vi "mono_rpm.vi"(7 "Sensor Connections":T1(array[cluster])) -> (0 "error out":errorcluster, 1 "wheel_rpm_sample":T2, 2 "Sensor Connections Out":T1(array[cluster]), 3 "tcp_out":refnum<k5>)   [LabVIEW 2018, in "monoDrive.lvlib"]
uses:
  monoDrive.lvlib
panel:
  in  "wheel_speed_rr":u8
  in  "wheel_speed_lr":u8
  in  "wheel_speed_rf":u8
  in  "wheel_speed_lf":u8
  in  "wheel_number":u32
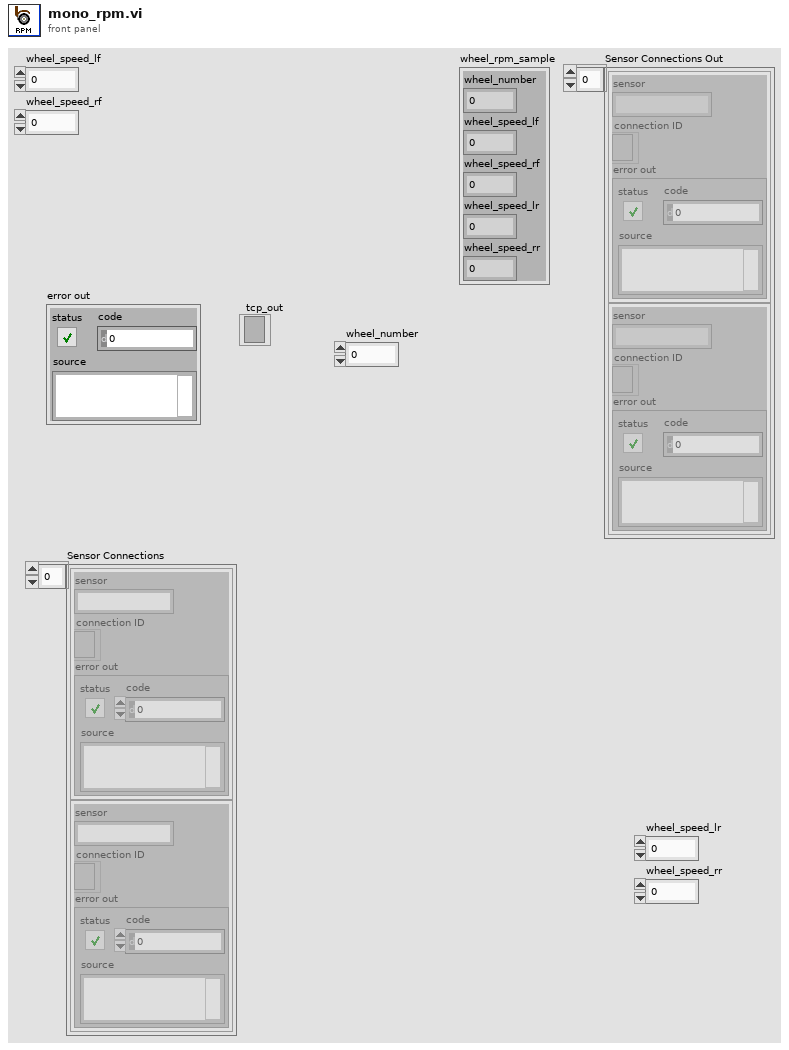
[diagram p1: front panel]
types:
  T1 = cluster{"sensor":string, "connection ID":refnum<k5>, "error out":errorcluster}[]
  T2 = cluster{"wheel_number":u32, "wheel_speed_lf":u8, "wheel_speed_rf":u8, "wheel_speed_lr":u8, "wheel_speed_rr":u8}
  T3 = cluster{"sensor":string, "connection ID":refnum<k5>, "error out":errorcluster}
  T4 = cluster{cluster{"length":u32, "time_stamp":u32, "game_time":sgl}, "data out":string}
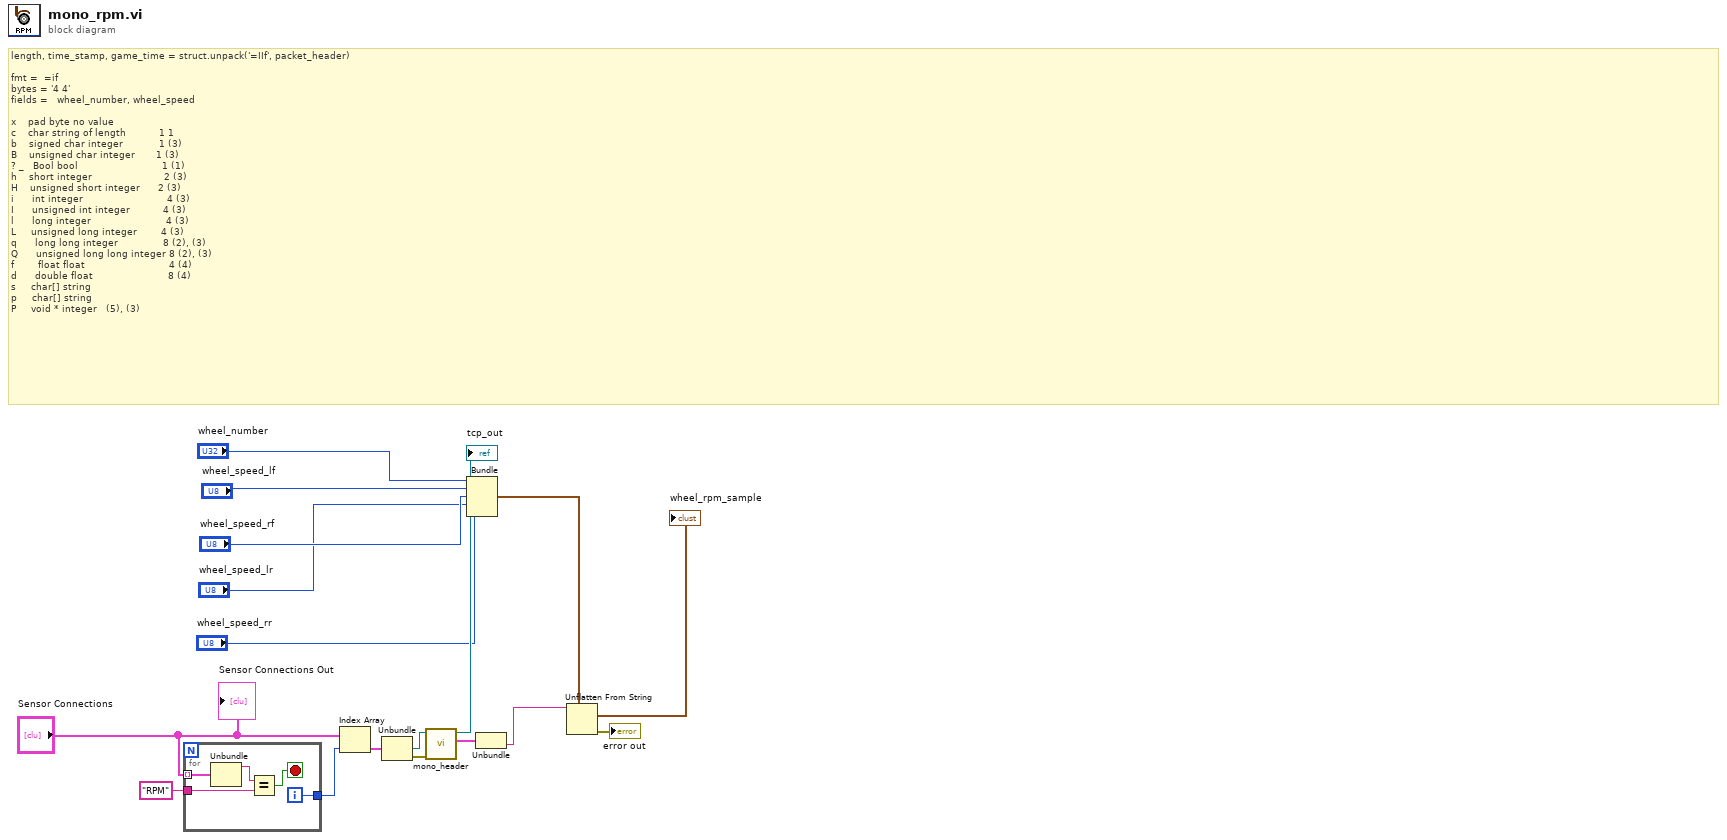
[diagram p0: block diagram]
diagram:
  # "length, time_stamp, game_time = struct.unpack('=IIf', packet_header)\n\nfmt =  =if\nbytes = '4 4'\nfields =   wheel_number, wheel_speed\n\nx\t   pad byte\tno value\t \t \nc\t   char\tstring of length           1\t1\t \nb\t   signed char\tinteger\t           1\t(3)\nB\t   unsigned char\tinteger\t      1\t(3)\n?\t_   Bool\tbool\t                           1\t(1)\nh\t   short\tinteger\t                       2\t(3)\nH\t   unsigned short\tinteger\t     2\t(3)\ni\t     int\tinteger\t                           4\t(3)\nI\t     unsigned int\tinteger\t          4\t(3)\nl     \tlong\tinteger\t                        4\t(3)\nL\t    unsigned long\tinteger\t       4\t(3)\nq     \tlong long\tinteger\t              8\t(2), (3)\nQ\t     unsigned long long\tinteger\t8\t(2), (3)\nf       \tfloat\tfloat\t                           4\t(4)\nd     \tdouble\tfloat\t                        8\t(4)\ns\t    char[]\tstring\t \t \np\t    char[]\tstring\t \t \nP\t    void *\tinteger\t \t(5), (3)"
  n1 = for {
    tunnel: "Sensor Connections" -> [w22] mode=indexing
    tunnel: "RPM" -> [w20]
    tunnel: [w18] -> w10
    i -> [w18]
    stop <- w19 stop-if-true
    n2 = Unbundle(w22) -> ("sensor"=w21:string)  [unwired: 2 out]
    n3 = Equal?(x=w21, y=w20) -> (x = y?=w19:bool)
  }
  n4 = Index Array(array="Sensor Connections", index=w10) -> (element=w14:T3)
  n5 = Unbundle(w14) -> ("connection ID"=w12:refnum<k5>, "error out"=w11:errorcluster)  [unwired: 1 out]
  n6 = call "mono_header.vi"("error in"=w11, "connection ID"=w12) -> ("sensor_sample"=w15:T4, "connection ID out"=→"tcp_out":refnum<k5>)  [unwired: 7 in, 1 out]
  n7 = Bundle("wheel_number"="wheel_number", "wheel_speed_lf"="wheel_speed_lf", "wheel_speed_rf"="wheel_speed_rf", "wheel_speed_lr"="wheel_speed_lr", "wheel_speed_rr"="wheel_speed_rr") -> (w17:T2)  [unwired: 1 in]
  n8 = Unbundle(w15) -> ("data out"=w6:string)  [unwired: 1 out]
  n9 = Unflatten From String(type=w17, binary string=w6) -> (value=→"wheel_rpm_sample":T2, error out=→"error out":errorcluster)  [unwired: 3 in, 1 out]
  "Sensor Connections Out" <- "Sensor Connections"
